vi "Continuous Counter.vi"(0 "value":u64, 1 "initial (0)":u64) -> (5 "count":u64)   [LabVIEW 2013]
doc: "This SubVI functions as a counter by adding the previous input to the current input. The counter can be initalized to a non-zero value."
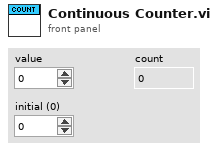
[diagram p1: front panel]
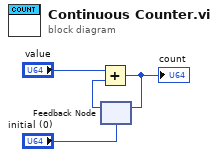
[diagram p0: block diagram]
diagram:
  n1 = feedback #1("initial (0)") -> (w3:u64)
  n2 = Add(x="value", y=w3) -> (x+y=w2:u64)
  "count" <- w2
  n3 = feedback-in #1(w2) -> ()
